vi "AH Read C and L.vi"(8 "Error In":errorcluster, 11 "VISA resource name":refnum<visa-resource-name>) -> (0 "Error Out":errorcluster, 1 "Loss":dbl, 2 "Capacitance":dbl, 3 "VISA resource name out":refnum<visa-resource-name>)   [LabVIEW 2016]
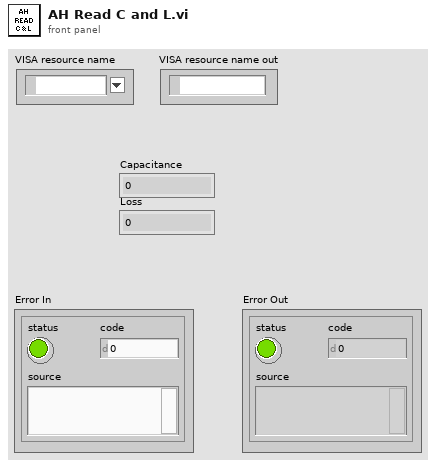
[diagram p1: front panel]
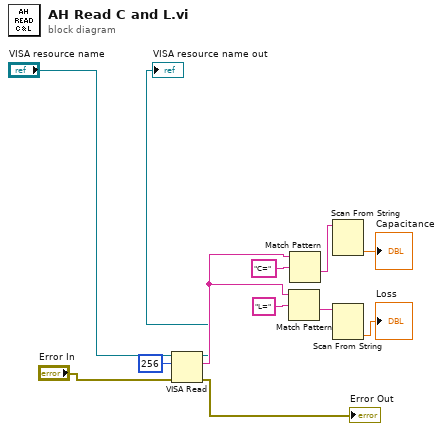
[diagram p0: block diagram]
diagram:
  n1 = VISA Read(VISA resource name="VISA resource name", byte count=u32 256, error in (no error)="Error In") -> (VISA resource name out=→"VISA resource name out":refnum<visa-resource-name>, read buffer=w4:string, error out=→"Error Out":errorcluster)  [unwired: 1 out]
  n2 = Match Pattern(string=w4, regular expression="L=") -> (after substring=w8:string)  [unwired: 4 out]
  n3 = Match Pattern(string=w4, regular expression="C=") -> (after substring=w11:string)  [unwired: 4 out]
  n4 = Scan From String(input string=w11) -> (output 1=→"Capacitance":dbl)  [unwired: 3 in, 4 out]
  n5 = Scan From String(input string=w8) -> (output 1=→"Loss":dbl)  [unwired: 3 in, 4 out]
